vi "Modificar_Entorno(SubVi).vi"(0 "Escala":dbl[][](array[numeric])=[[1.0, 1.0, 1.0], [1.0, 1.0, 1.0], [1.0, 1.0, 1.0]], 1 "Translación":dbl[][](array[numeric])=[[1.0, 1.0, 0.0], [0.0, 0.0, 0.0], [0.0, 0.0, 0.0]], 2 "Rotación":dbl[][](array[numeric])=[[1.0, 0.0, 0.0, 0.0], [1.0, 0.0, 0.0, 0.0], [1.0, 0.0, 0.0, 0.0]], 3 "Operación":T3, 4 "Eje de la Figura":T2, 5 "Figura Geometrica":T1, 7 "Valor":dbl format="%#_13g") -> (14 "Escala Salida":dbl[][](array[numeric]), 15 "Translación Salida":dbl[][](array[numeric]), 16 "Rotación Salida":dbl[][](array[numeric]))   [LabVIEW 2017]
uses:
  Control_Operacion.ctl
  Control_Eje_Figura.ctl
  Control_Figura.ctl
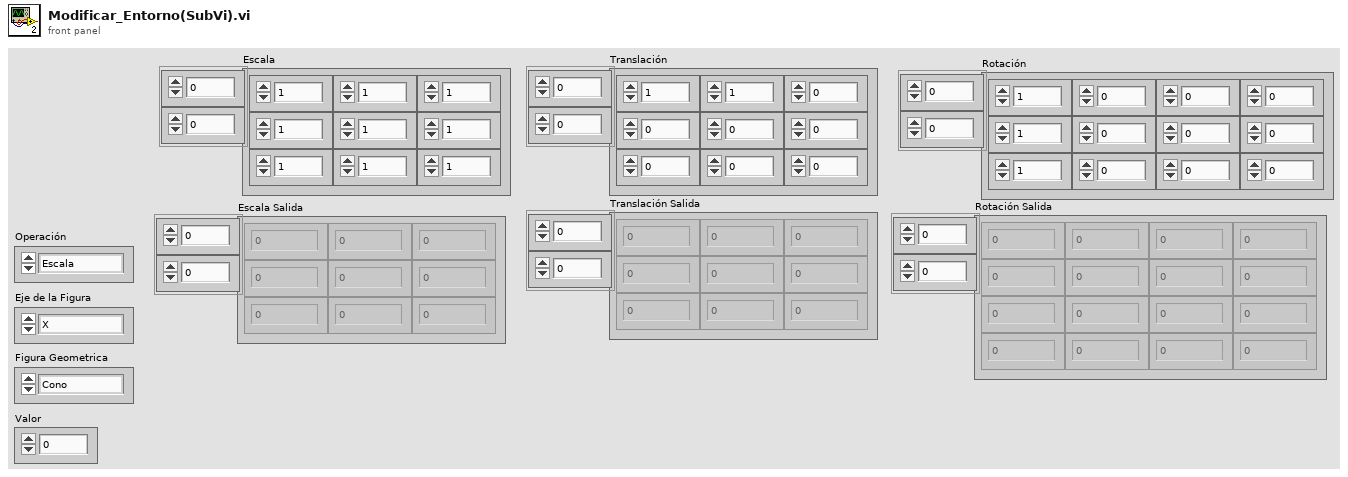
[diagram p1: front panel]
types:
  T1 = typedef "Control_Figura.ctl" = enum16{"Cono", "Esfera", "Cilindro"}
  T2 = typedef "Control_Eje_Figura.ctl" = enum16{"X", "Y", "Z"}
  T3 = typedef "Control_Operacion.ctl" = enum16{"Escala", "Translación", "Rotación"}
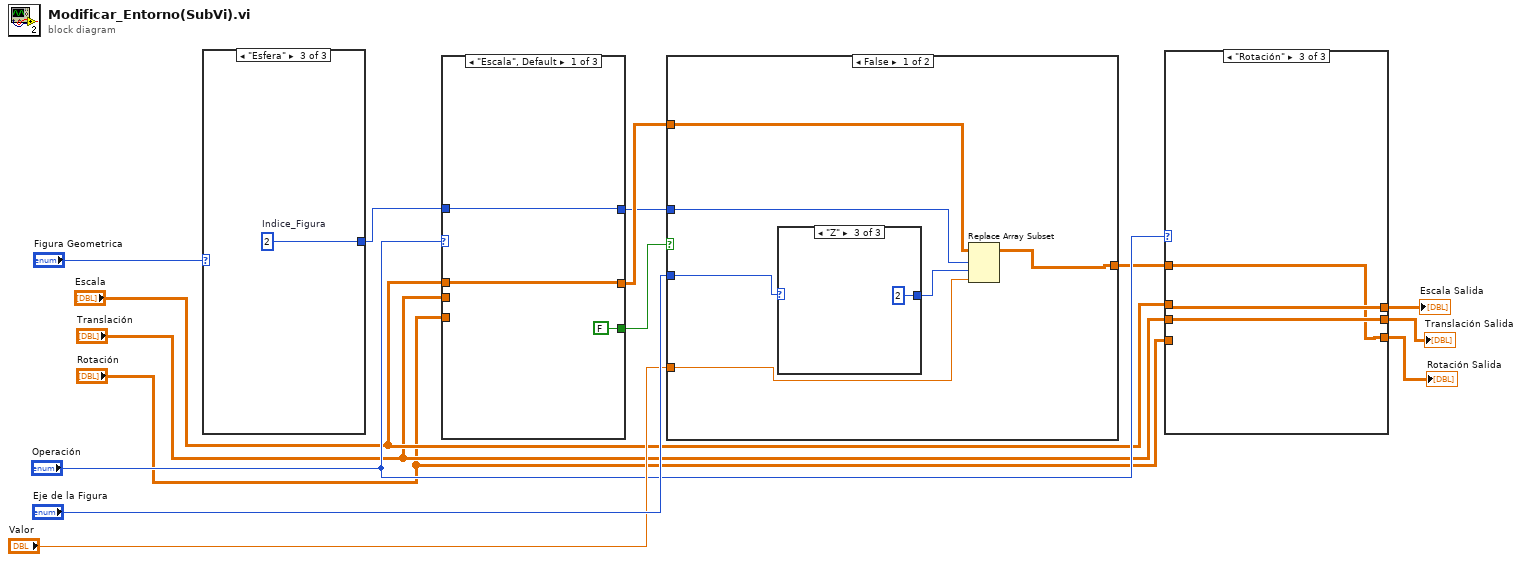
[diagram p0: block diagram]
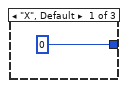
[diagram p4: hidden frame]
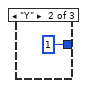
[diagram p5: hidden frame]
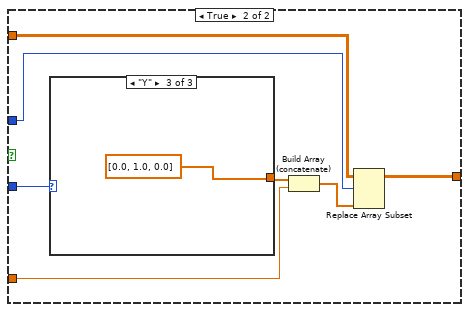
[diagram p6: hidden frame]
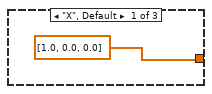
[diagram p7: hidden frame]
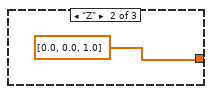
[diagram p8: hidden frame]
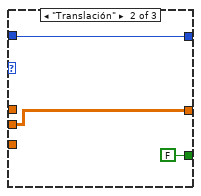
[diagram p9: hidden frame]
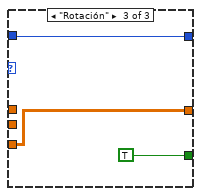
[diagram p10: hidden frame]
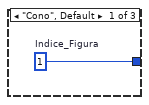
[diagram p11: hidden frame]
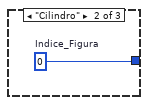
[diagram p12: hidden frame]
diagram:
  n1 = case shown="\"Esfera\"" "Figura Geometrica" {
    tunnel: [w16 w17 w18] -> w14
    frame "Cono", Default {
      w16 = 1  # Indice_Figura
    }
    frame "Cilindro" {
      w17 = 0  # Indice_Figura
    }
    frame "Esfera" {
      w18 = 2  # Indice_Figura
    }
  }
  n2 = case shown="\"Escala\", Default" "Operación" {
    tunnel: "Escala" -> [w21 _ _]
    tunnel: "Translación" -> [_ w23 _]
    tunnel: "Rotación" -> [_ _ w27]
    tunnel: w14 -> [w20 w24 w26]
    tunnel: [w21 w23 w27] -> w10
    tunnel: [w20 w24 w26] -> w9
    tunnel: [FALSE FALSE TRUE] -> w13
    frame "Escala", Default {
    }
    frame "Translación" {
    }
    frame "Rotación" {
    }
  }
  n3 = case shown="False" w13 {
    tunnel: "Eje de la Figura" -> [w31 w43]
    tunnel: "Valor" -> [w29 w41]
    tunnel: w10 -> [w33 w40]
    tunnel: w9 -> [w32 w39]
    tunnel: [w28 w37] -> w7
    frame False {
      n4 = case shown="\"Z\"" w31 {
        tunnel: [0 1 2] -> w30
        frame "X", Default {
        }
        frame "Y" {
        }
        frame "Z" {
        }
      }
      n5 = Replace Array Subset(array=w33, new element=w29, index (row)=w32, index (col)=w30) -> (w28:dbl[][])
    }
    frame True {
      n6 = case shown="\"Y\"" w43 {
        tunnel: [dbl[] [1.0, 0.0, 0.0] dbl[] [0.0, 0.0, 1.0] dbl[] [0.0, 1.0, 0.0]] -> w42
        frame "X", Default {
        }
        frame "Z" {
        }
        frame "Y" {
        }
      }
      n7 = Build Array (concatenate)(w42, w41) -> (w38:dbl[])
      n8 = Replace Array Subset(array=w40, new element=w38, index (row)=w39) -> (w37:dbl[][])  [unwired: 1 in]
    }
  }
  n9 = case shown="\"Rotación\"" "Operación" {
    tunnel: w7 -> [w47 w50 w53]
    tunnel: "Escala" -> [_ w52 w54]
    tunnel: "Translación" -> [w49 _ w55]
    tunnel: "Rotación" -> [w48 w51 _]
    tunnel: [w49 w50 w55] -> w2
    tunnel: [w48 w51 w53] -> w1
    tunnel: [w47 w52 w54] -> w3
    frame "Escala", Default {
    }
    frame "Translación" {
    }
    frame "Rotación" {
    }
  }
  "Escala Salida" <- w3
  "Translación Salida" <- w2
  "Rotación Salida" <- w1
